vi "ErrorHandler.vi"(8 "错误输入（无错误）":errorcluster, 11 "Execute输入":refnum<class "Execute.lvclass">) -> (0 "错误输出":errorcluster, 3 "Execute输出":refnum<class "Execute.lvclass">)   [LabVIEW 2018, in "QMH_Class.lvlib" / "TestManager.lvlib" / "Execute.lvclass"]
uses:
  Execute.lvclass
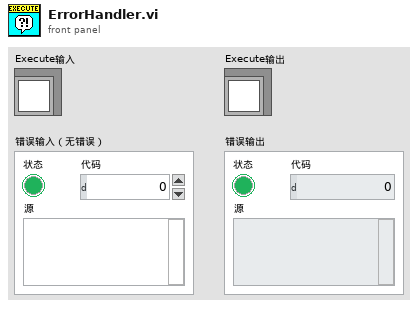
[diagram p1: front panel]
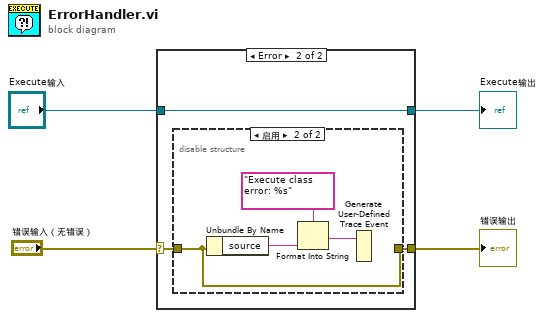
[diagram p0: block diagram]
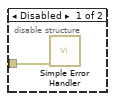
[diagram p3: hidden frame]
diagram:
  n1 = case shown="Error" "错误输入（无错误）" {
    selector: "错误输入（无错误）" -> [w5 w8]
    tunnel: [w6 w9] -> w1
    tunnel: "Execute输入" -> [w6 w9]
    tunnel: [w5 w7] -> w2
    frame No Error {
    }
    frame Error {
      n2 = disable-structure shown="启用" {
        disable-tunnel: w8 -> [w10 w11]
        disable-tunnel: [_ w11] -> w7
        frame Disabled {
          n3 = call <vilib>:"Simple Error Handler.vi"("error in (no error)"=w10) -> ()  [unwired: 4 in, 5 out]
        }
        frame Enabled {
          n4 = Unbundle By Name(w11) -> ("source"=w14:string)
          n5 = Format Into String(format string="Execute class error: %s" ("格式字符串"), w14) -> (resulting string=w13:string)  [unwired: 2 in, 1 out]
          n6 = Generate User-Defined Trace Event(2:w13) -> ()  [unwired: 1 in]
        }
      }
    }
  }
  "错误输出" <- w2
  "Execute输出" <- w1
